vi "Move XYA.vi"(3 "Make Vertical":bool, 4 "Side":T1=enum."right", 5 "Label":string, 6 "Wait Time":dbl, 8 "error in":errorcluster, 9 "Speed (mm/s)":dbl=50.0, 10 "XYA":cluster{"X":dbl, "Y":dbl, "A":dbl}, 11 "Location":string="Current") -> (0 "error out":errorcluster)   [LabVIEW 2013]
uses:
  ROS/Code/SubVIs/BaxterSide.ctl
  Move XYZA.vi
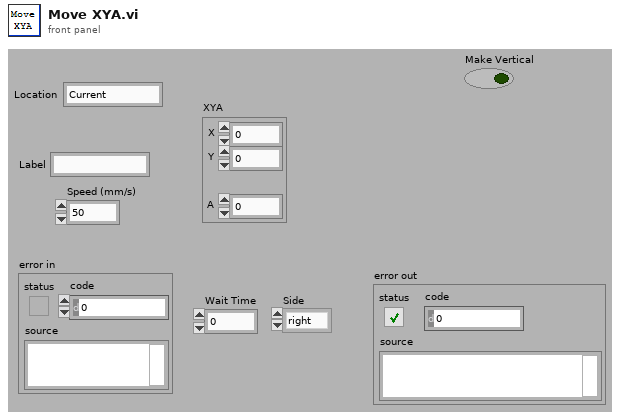
[diagram p1: front panel]
types:
  T1 = typedef "BaxterSide.ctl" = enum16{"left", "right"}
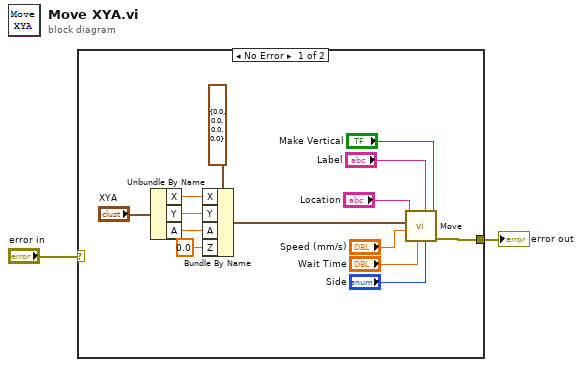
[diagram p0: block diagram]
diagram:
  n1 = case shown="No Error" "error in" {
    selector: "error in" -> [_ w17]
    tunnel: [w15 w17] -> w1
    frame No Error {
      n2 = Unbundle By Name("XYA") -> ("X"=w10:dbl, "Y"=w11:dbl, "A"=w12:dbl)
      n3 = Bundle By Name(cluster=cluster{"X":dbl, "Y":dbl, "Z":dbl, "A":dbl} {"X"=0.0, "Y"=0.0, "Z"=0.0, "A"=0.0} ("XYZA"), "X"=w10, "Y"=w11, "A"=w12, "Z"=0.0) -> (w7:cluster{"X":dbl, "Y":dbl, "Z":dbl, "A":dbl})
      n4 = call-poly "Move.vi"("Make Vertical"="Make Vertical", "Side"="Side", "Label"="Label", "Wait Time"="Wait Time", "Speed (mm/s)"="Speed (mm/s)", "XYZA"=w7, "Location"="Location") -> ("error out"=w15:errorcluster)  [unwired: 4 in]
    }
    frame Error {
    }
  }
  "error out" <- w1
